vi "Configure Instrument.vi"(8 "error in (no error)":errorcluster, 11 "Example Instrument in":refnum<class "Example.lvclass">) -> (0 "error out":errorcluster, 3 "Example Instrument out":refnum<class "Example.lvclass">)   [LabVIEW 2019, in "Example.lvclass"]
uses:
  Example.lvclass
  Instrument Types/VSource/Instrument.VSource.lvclass
panel:
  # "Use this if you want to \nhave a configuration\nwindow specific to your\ninstrument. Otherwise you\nmay delete"
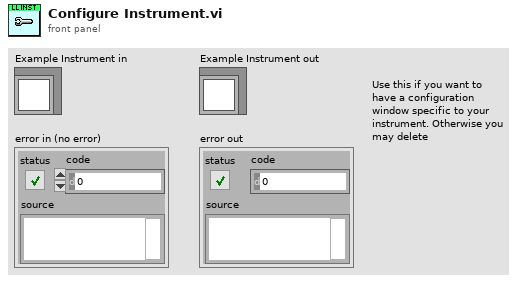
[diagram p1: front panel]
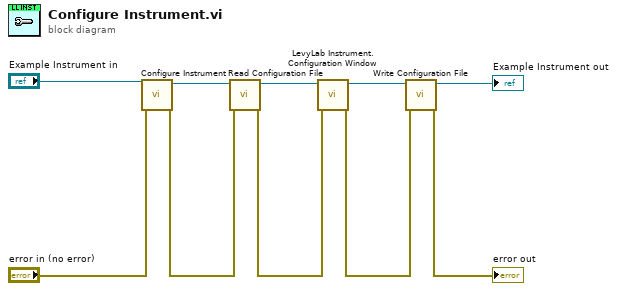
[diagram p0: block diagram]
diagram:
  n1 = call-parent "Configure Instrument.vi"("error in (no error)"="error in (no error)", "Instrument in"="Example Instrument in") -> ("error out"=w5:errorcluster, "Instrument out"=w7:refnum<class "Example.lvclass">)  [unwired: 8 in]
  n2 = call-dynamic "Read Configuration File.vi"("error in (no error)"=w5, "Example Instrument in"=w7) -> ("error out"=w4:errorcluster, "Example Instrument out"=w3:refnum<class "Example.lvclass">)  [unwired: 8 in]
  n3 = call "LevyLab Instrument.Configuration Window.vi"("error in (no error)"=w4, "Example Instrument in"=w3) -> ("error out"=w1:errorcluster, "Example Instrument out"=w2:refnum<class "Example.lvclass">)  [unwired: 8 in]
  n4 = call-dynamic "Write Configuration File.vi"("error in (no error)"=w1, "Example Instrument in"=w2) -> ("error out"=→"error out":errorcluster, "Example Instrument out"=→"Example Instrument out":refnum<class "Example.lvclass">)  [unwired: 8 in]
